vi "Log GV.vi"() -> ()   [LabVIEW 2019, in "Log.lvlib"]
uses:
  Log.lvlib
  log module message.ctl
  mmw_command_lib/src_LabVIEW/mmW_commands/TypeDefs/commands.ctl
  mmw_command_lib/src_LabVIEW/mmW_commands/mmW_commands.lvlib
panel:
  in  "time.fetch":dbl format="%#_6p"
  in  "time.send_trig":dbl format="%#_6p"
  in  "time.start":dbl format="%#_6p"
  in  "time.config_rf":dbl format="%#_6p"
  in  "time.initialize_hw":dbl format="%#_6p"
  out "Execution benchmark":cluster{"command out":T1, "final time":dbl}[](array[cluster]) {"final time" format="%#_6p"}
  in  "Log event":refnum<user-event>
  in  "Debug log":string[][](array[string])
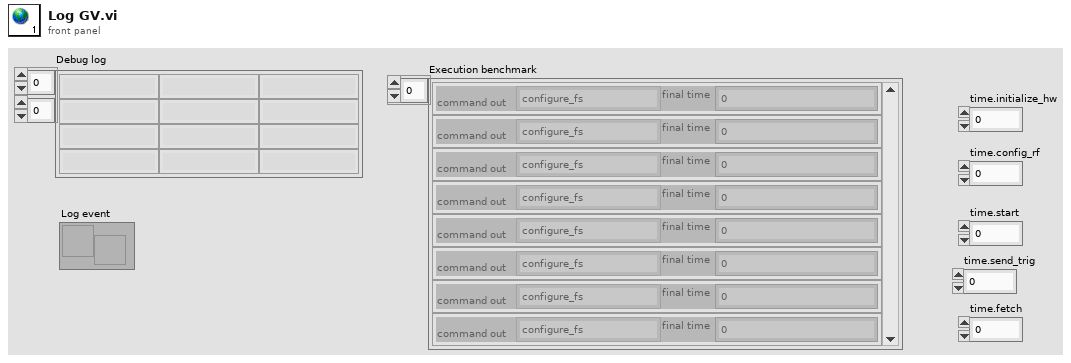
[diagram p1: front panel]
types:
  T1 = typedef "mmW_commands.lvlib/commands.ctl" = enum16{"configure_fs", "configure_rf", "configure_trigger", "equalization_enable", "equalization_start", "lo_sync_enable", "equalization_stop", "get_instrument_status", "get_versions", "initialize_hw", "pop_rx", "set_log_level", "Shutdown", "start", "start_instrument_app", "stop", "trans", "transceive", "trigger_burst", "trigger_sync_enable", "Write TX", "resp_generic", "resp_waveform", "send_trigger", "fetch", "transceive2"}
diagram:
